vi "AGGIUNGI CARATTERISTICHE GRAFICO.vi"() -> ()   [LabVIEW 2019]
uses:
  TypeDef/Definizione_Grafico_REPORT_OLD.ctl
  TypeDef/Definizione_Grafico_REPORT.ctl
panel:
  out "output cluster":T1={"ASSE X 1"={"NOME ASSE"="", "AUTO\nSCALA?"=FALSE, "MIN"=0.0, "MAX"=0.0, "Colore asse"=0, "Griglie Maggiori"=0, "Griglie Minori"=0, "Decimali"=1}, "ASSE X 2"={"NOME ASSE"="", "AUTO\nSCALA?"=FALSE, "MIN"=0.0, "MAX"=0.0, "Colore asse"=0, "Griglie Maggiori"=0, "Griglie Minori"=0, "Decimali"=1}, "ASSE Y 1"={"NOME ASSE"="", "AUTO\nSCALA?"=FALSE, "MIN"=0.0, "MAX"=0.0, "Colore asse"=0, "Griglie Maggiori"=0, "Griglie Minori"=0, "Decimali"=1}, "ASSE Y 2"={"NOME ASSE"="", "AUTO\nSCALA?"=FALSE, "MIN"=0.0, "MAX"=0.0, "Colore asse"=0, "Griglie Maggiori"=0, "Griglie Minori"=0, "Decimali"=1}, "ASSE Y 3"={"NOME ASSE"="", "AUTO\nSCALA?"=FALSE, "MIN"=0.0, "MAX"=0.0, "Colore asse"=0, "Griglie Maggiori"=0, "Griglie Minori"=0, "Decimali"=1}, "ASSE Y 4"={"NOME ASSE"="", "AUTO\nSCALA?"=FALSE, "MIN"=0.0, "MAX"=0.0, "Colore asse"=0, "Griglie Maggiori"=0, "Griglie Minori"=0, "Decimali"=1}, "X1"=FALSE, "X2"=FALSE, "Y1"=FALSE, "Y2"=FALSE, "Y3"=FALSE, "Y4"=FALSE, "NOME GRAFICO"="", "PROVE ASSOCIATE"={"A FREDDO"=FALSE, "A VUOTO"=FALSE, "A CARICO"=FALSE, "TERMICA"=FALSE, "C.MECC."=FALSE, "ROT BLOCC"=FALSE, "GENERICA"=FALSE, "TABELLA RESISTOMAT"=FALSE, "SCORTA 2"=FALSE, "SCORTA 3"=FALSE}, "ASSE Y 5"={"NOME ASSE"="", "AUTO\nSCALA?"=FALSE, "MIN"=0.0, "MAX"=0.0, "Colore asse"=0, "Griglie Maggiori"=0, "Griglie Minori"=0, "Decimali"=1}, "Y5"=FALSE, "Colore sfondo grafico"=0} {"ASSE Y 5"."Decimali" min=0; "ASSE Y 4"."Decimali" min=0; "ASSE Y 3"."Decimali" min=0; "ASSE Y 2"."Decimali" min=0; "ASSE Y 1"."Decimali" min=0; "ASSE X 2"."Decimali" min=0; "ASSE X 1"."Decimali" min=0}
  in  "file path (use dialog)":path
  out "GRAFICO":T2={"ASSE X 1"={"NOME ASSE"="Time[s]", "AUTO\nSCALA?"=TRUE, "MIN"=0.0, "MAX"=0.0, "Colore asse"=16448250, "Griglie Maggiori"=0, "Griglie Minori"=0}, "ASSE X 2"={"NOME ASSE"="", "AUTO\nSCALA?"=FALSE, "MIN"=0.0, "MAX"=0.0, "Colore asse"=16448250, "Griglie Maggiori"=0, "Griglie Minori"=0}, "ASSE Y 1"={"NOME ASSE"="Voltage[V]", "AUTO\nSCALA?"=TRUE, "MIN"=0.0, "MAX"=0.0, "Colore asse"=16448250, "Griglie Maggiori"=0, "Griglie Minori"=0}, "ASSE Y 2"={"NOME ASSE"="C[Nm]", "AUTO\nSCALA?"=FALSE, "MIN"=0.0, "MAX"=1.0, "Colore asse"=16448250, "Griglie Maggiori"=0, "Griglie Minori"=0}, "ASSE Y 3"={"NOME ASSE"="Pot[kW]", "AUTO\nSCALA?"=FALSE, "MIN"=0.0, "MAX"=0.0, "Colore asse"=16448250, "Griglie Maggiori"=0, "Griglie Minori"=0}, "ASSE Y 4"={"NOME ASSE"="eff[%]", "AUTO\nSCALA?"=FALSE, "MIN"=0.0, "MAX"=0.0, "Colore asse"=16448250, "Griglie Maggiori"=0, "Griglie Minori"=0}, "X1"=TRUE, "X2"=FALSE, "Y1"=TRUE, "Y2"=TRUE, "Y3"=FALSE, "Y4"=FALSE, "NOME GRAFICO"="Voltage-Time 2", "PROVE ASSOCIATE"={"A FREDDO"=FALSE, "A VUOTO"=TRUE, "A CARICO"=FALSE, "TERMICA"=FALSE, "C.MECC."=FALSE, "ROT BLOCC"=FALSE, "GENERICA"=FALSE, "SCORTA 1"=FALSE, "SCORTA 2"=FALSE, "SCORTA 3"=FALSE}, "ASSE Y 5"={"NOME ASSE"="", "AUTO\nSCALA?"=FALSE, "MIN"=0.0, "MAX"=0.0, "Colore asse"=16448250, "Griglie Maggiori"=0, "Griglie Minori"=0}, "Y5"=FALSE, "Colore sfondo grafico"=0}
  out "Array":T2[](array[typedef])
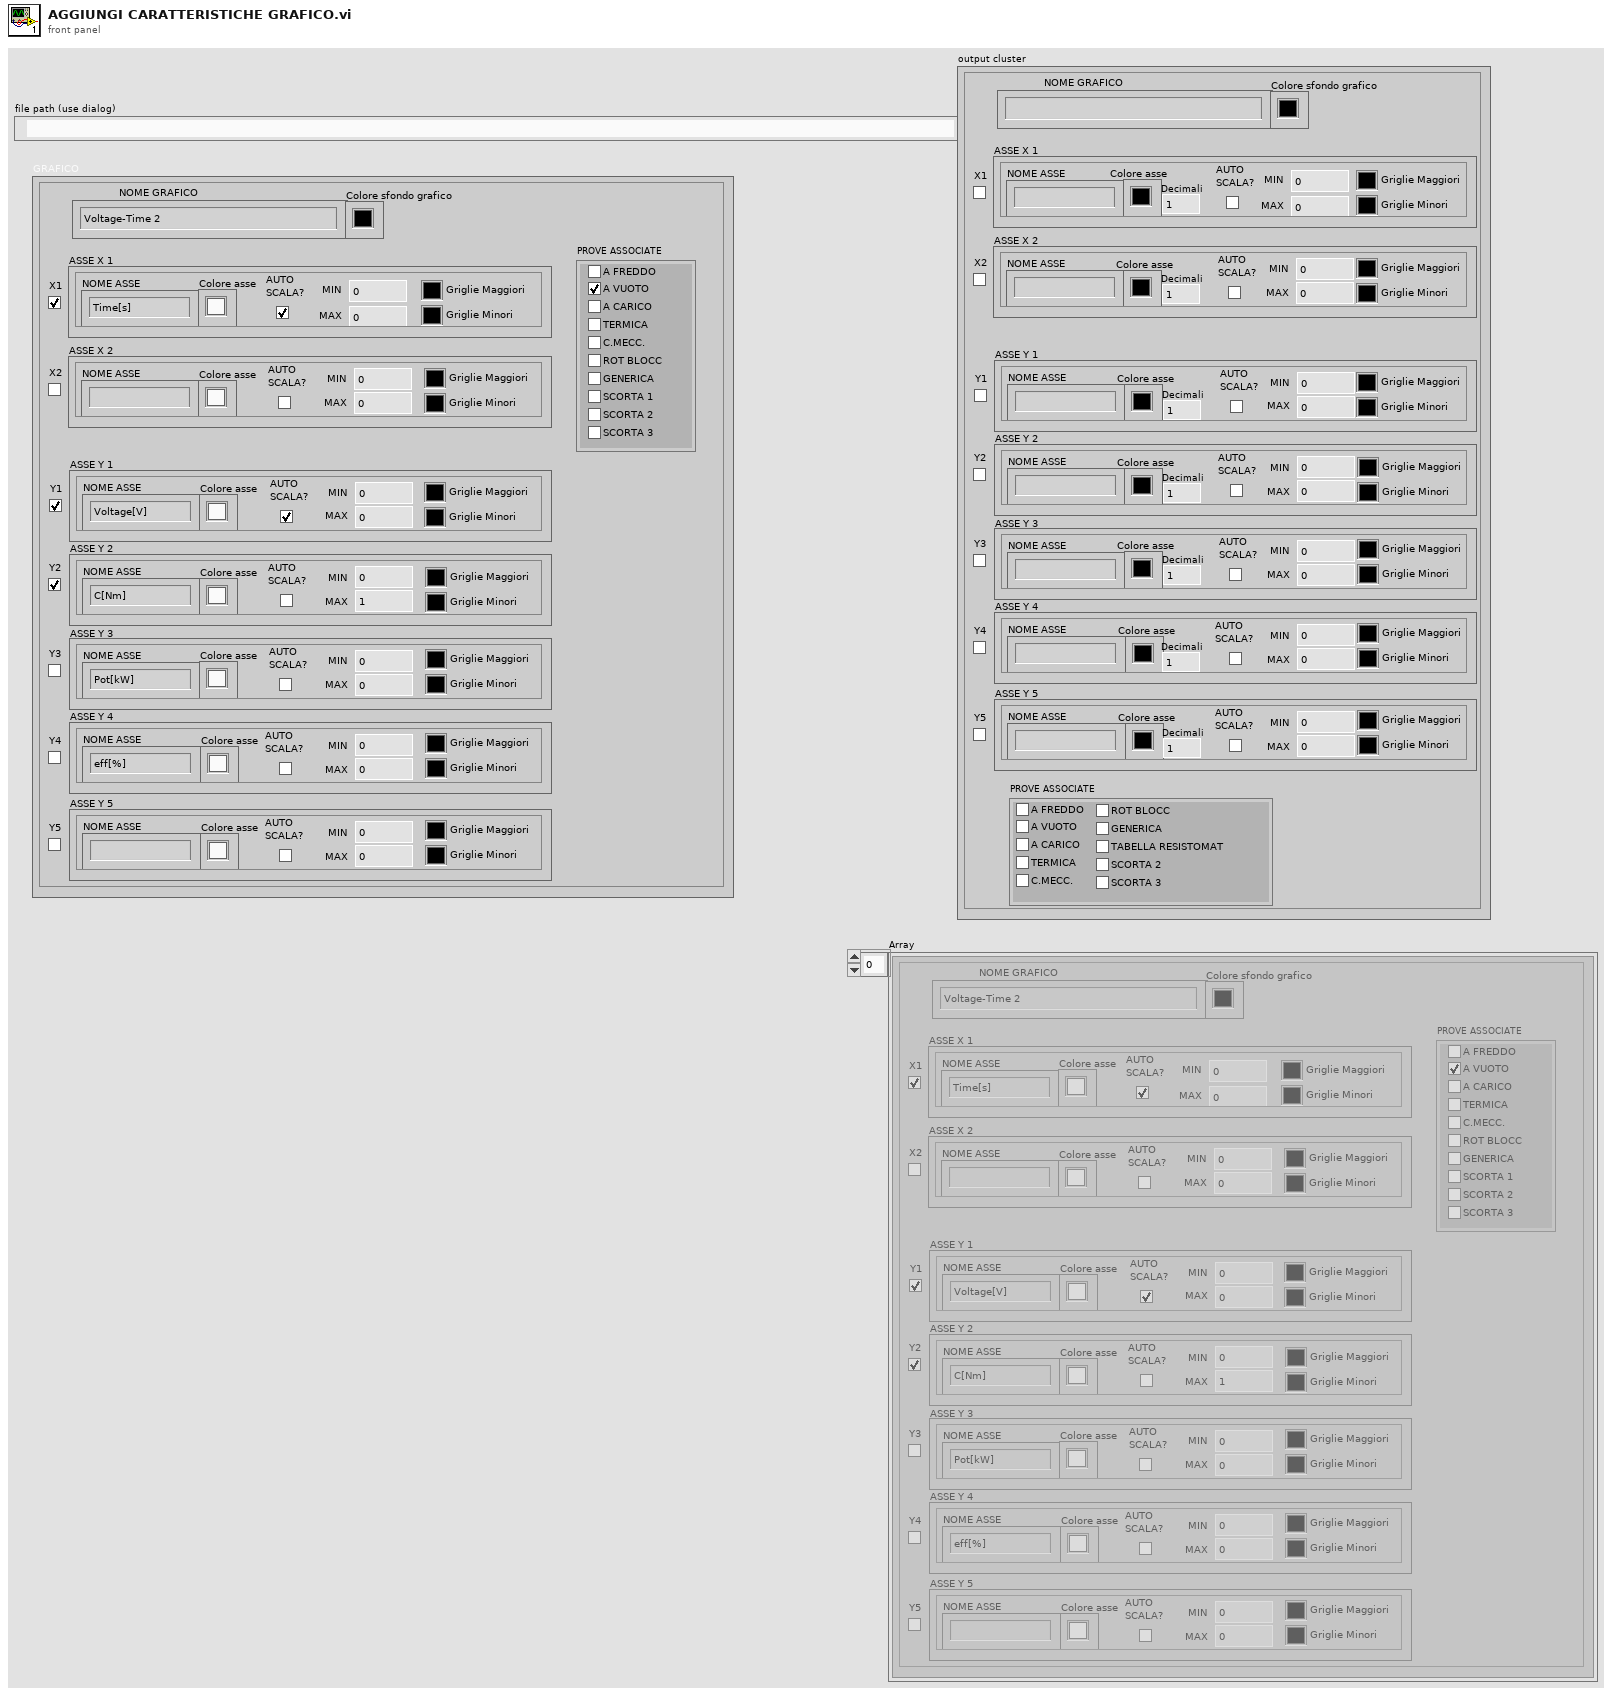
[diagram p1: front panel]
types:
  T1 = typedef "Definizione_Grafico_REPORT.ctl" = cluster{"ASSE X 1":cluster{"NOME ASSE":string, "AUTO\nSCALA?":bool, "MIN":dbl, "MAX":dbl, "Colore asse":u32, "Griglie Maggiori":u32, "Griglie Minori":u32, "Decimali":i8}, "ASSE X 2":cluster{"NOME ASSE":string, "AUTO\nSCALA?":bool, "MIN":dbl, "MAX":dbl, "Colore asse":u32, "Griglie Maggiori":u32, "Griglie Minori":u32, "Decimali":i8}, "ASSE Y 1":cluster{"NOME ASSE":string, "AUTO\nSCALA?":bool, "MIN":dbl, "MAX":dbl, "Colore asse":u32, "Griglie Maggiori":u32, "Griglie Minori":u32, "Decimali":i8}, "ASSE Y 2":cluster{"NOME ASSE":string, "AUTO\nSCALA?":bool, "MIN":dbl, "MAX":dbl, "Colore asse":u32, "Griglie Maggiori":u32, "Griglie Minori":u32, "Decimali":i8}, "ASSE Y 3":cluster{"NOME ASSE":string, "AUTO\nSCALA?":bool, "MIN":dbl, "MAX":dbl, "Colore asse":u32, "Griglie Maggiori":u32, "Griglie Minori":u32, "Decimali":i8}, "ASSE Y 4":cluster{"NOME ASSE":string, "AUTO\nSCALA?":bool, "MIN":dbl, "MAX":dbl, "Colore asse":u32, "Griglie Maggiori":u32, "Griglie Minori":u32, "Decimali":i8}, "X1":bool, "X2":bool, "Y1":bool, "Y2":bool, "Y3":bool, "Y4":bool, "NOME GRAFICO":string, "PROVE ASSOCIATE":cluster{"A FREDDO":bool, "A VUOTO":bool, "A CARICO":bool, "TERMICA":bool, "C.MECC.":bool, "ROT BLOCC":bool, "GENERICA":bool, "TABELLA RESISTOMAT":bool, "SCORTA 2":bool, "SCORTA 3":bool}, "ASSE Y 5":cluster{"NOME ASSE":string, "AUTO\nSCALA?":bool, "MIN":dbl, "MAX":dbl, "Colore asse":u32, "Griglie Maggiori":u32, "Griglie Minori":u32, "Decimali":i8}, "Y5":bool, "Colore sfondo grafico":u32}
  T2 = typedef "Definizione_Grafico_REPORT_OLD.ctl" = cluster{"ASSE X 1":cluster{"NOME ASSE":string, "AUTO\nSCALA?":bool, "MIN":dbl, "MAX":dbl, "Colore asse":u32, "Griglie Maggiori":u32, "Griglie Minori":u32}, "ASSE X 2":cluster{"NOME ASSE":string, "AUTO\nSCALA?":bool, "MIN":dbl, "MAX":dbl, "Colore asse":u32, "Griglie Maggiori":u32, "Griglie Minori":u32}, "ASSE Y 1":cluster{"NOME ASSE":string, "AUTO\nSCALA?":bool, "MIN":dbl, "MAX":dbl, "Colore asse":u32, "Griglie Maggiori":u32, "Griglie Minori":u32}, "ASSE Y 2":cluster{"NOME ASSE":string, "AUTO\nSCALA?":bool, "MIN":dbl, "MAX":dbl, "Colore asse":u32, "Griglie Maggiori":u32, "Griglie Minori":u32}, "ASSE Y 3":cluster{"NOME ASSE":string, "AUTO\nSCALA?":bool, "MIN":dbl, "MAX":dbl, "Colore asse":u32, "Griglie Maggiori":u32, "Griglie Minori":u32}, "ASSE Y 4":cluster{"NOME ASSE":string, "AUTO\nSCALA?":bool, "MIN":dbl, "MAX":dbl, "Colore asse":u32, "Griglie Maggiori":u32, "Griglie Minori":u32}, "X1":bool, "X2":bool, "Y1":bool, "Y2":bool, "Y3":bool, "Y4":bool, "NOME GRAFICO":string, "PROVE ASSOCIATE":cluster{"A FREDDO":bool, "A VUOTO":bool, "A CARICO":bool, "TERMICA":bool, "C.MECC.":bool, "ROT BLOCC":bool, "GENERICA":bool, "SCORTA 1":bool, "SCORTA 2":bool, "SCORTA 3":bool}, "ASSE Y 5":cluster{"NOME ASSE":string, "AUTO\nSCALA?":bool, "MIN":dbl, "MAX":dbl, "Colore asse":u32, "Griglie Maggiori":u32, "Griglie Minori":u32}, "Y5":bool, "Colore sfondo grafico":u32}
  T3 = enum16{"open", "replace", "create", "open or create", "replace or create", "replace or create with confirmation"}
  T4 = cluster{"A FREDDO":bool, "A VUOTO":bool, "A CARICO":bool, "TERMICA":bool, "C.MECC.":bool, "ROT BLOCC":bool, "GENERICA":bool, "SCORTA 1":bool, "SCORTA 2":bool, "SCORTA 3":bool}
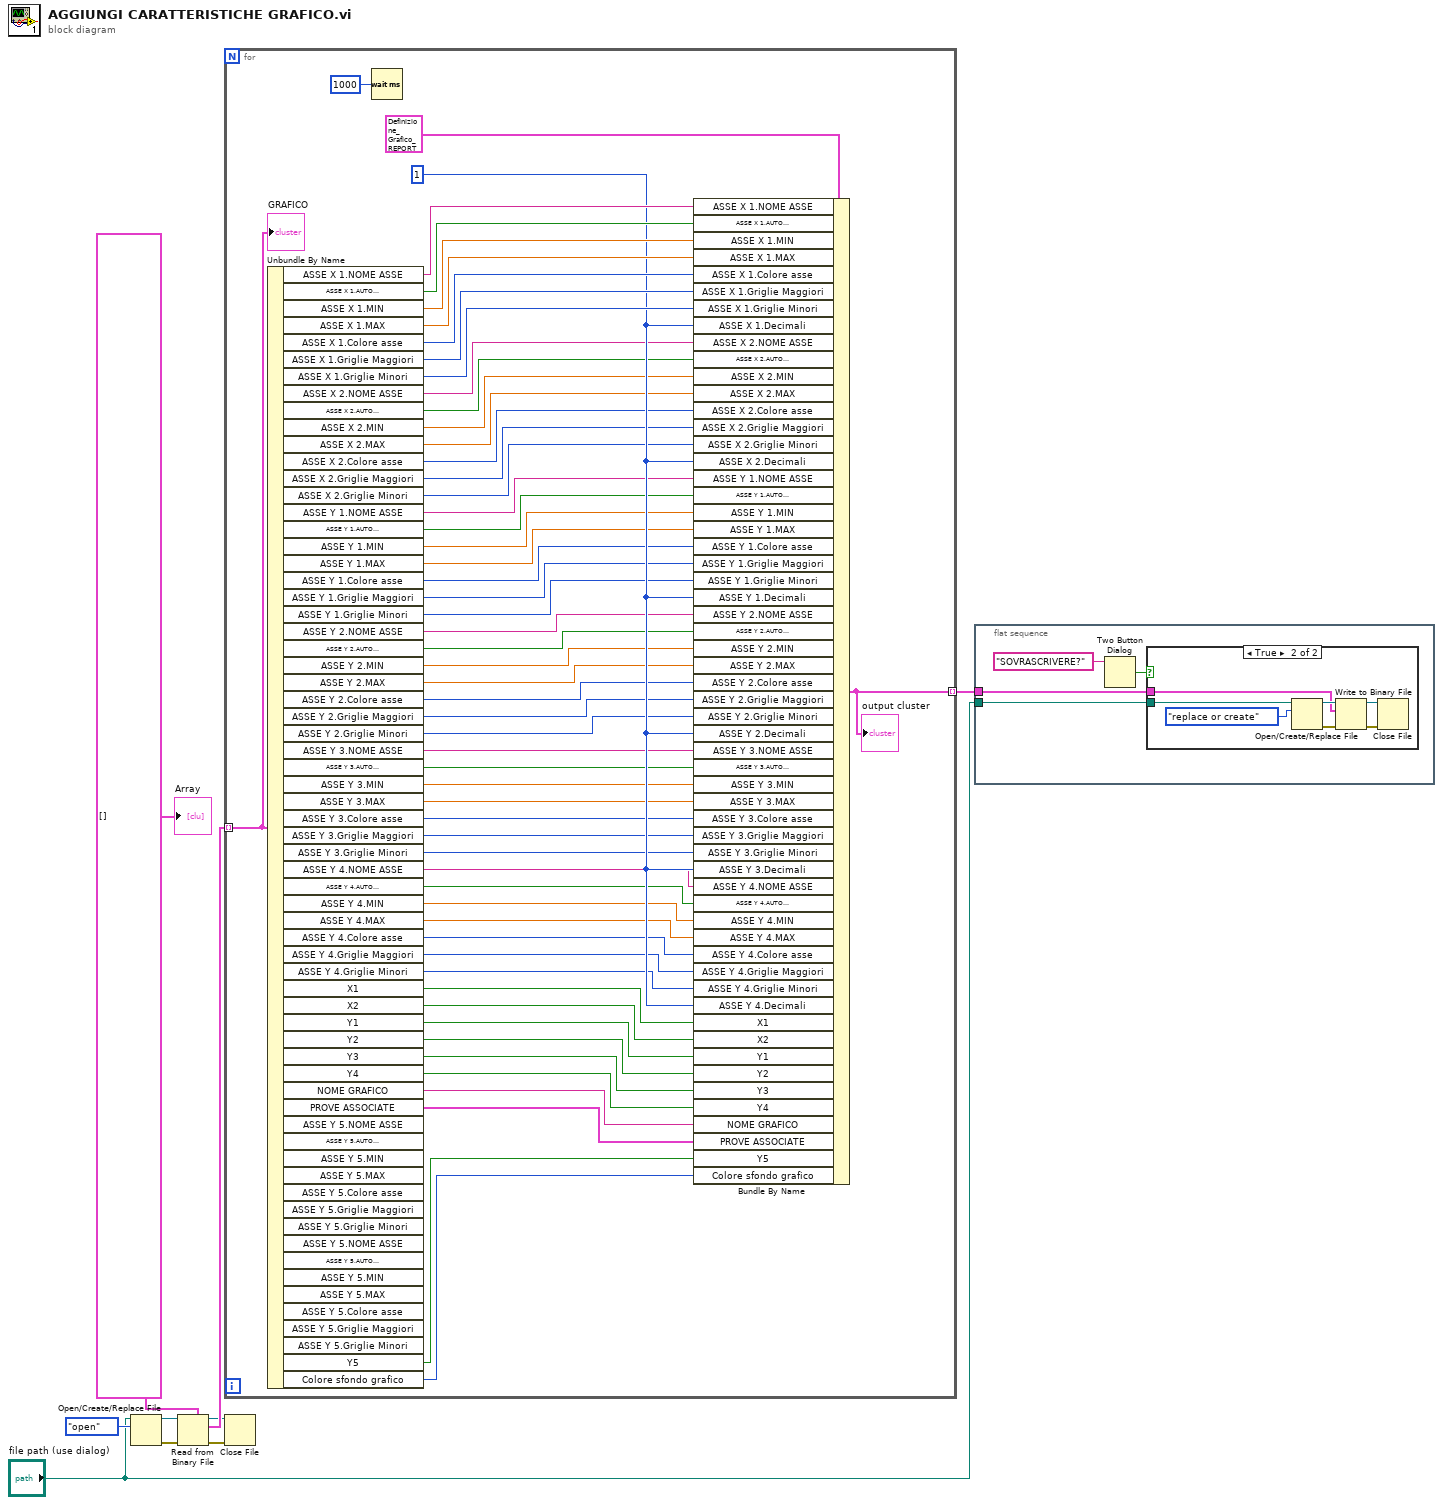
[diagram p0: block diagram]
diagram:
  w5 = T2[] []
  n1 = Open/Create/Replace File(file path (use dialog)="file path (use dialog)", operation (0:open)=T3."open") -> (refnum out=w8:refnum<file>, error out=w9:errorcluster)  [unwired: 4 in, 1 out]
  n2 = Read from Binary File(5:w5, 8:w9, 11:w8) -> (0:w3:errorcluster, 2:w6:T2[], 3:w4:refnum<file>)  [unwired: 3 in, 1 out]
  n3 = for {
    tunnel: w6 -> [w11] mode=indexing
    tunnel: [w12] -> w1 mode=indexing
    w58 = 1
    n4 = Unbundle By Name(w11) -> ("ASSE X 1.NOME ASSE"=w65:string, "ASSE X 1.AUTO\nSCALA?"=w64:bool, "ASSE X 1.MIN"=w63:dbl, "ASSE X 1.MAX"=w62:dbl, "ASSE X 1.Colore asse"=w61:u32, "ASSE X 1.Griglie Maggiori"=w60:u32, "ASSE X 1.Griglie Minori"=w59:u32, "ASSE X 2.NOME ASSE"=w57:string, "ASSE X 2.AUTO\nSCALA?"=w56:bool, "ASSE X 2.MIN"=w55:dbl, "ASSE X 2.MAX"=w54:dbl, "ASSE X 2.Colore asse"=w53:u32, "ASSE X 2.Griglie Maggiori"=w52:u32, "ASSE X 2.Griglie Minori"=w51:u32, "ASSE Y 1.NOME ASSE"=w50:string, "ASSE Y 1.AUTO\nSCALA?"=w49:bool, "ASSE Y 1.MIN"=w48:dbl, "ASSE Y 1.MAX"=w47:dbl, "ASSE Y 1.Colore asse"=w46:u32, "ASSE Y 1.Griglie Maggiori"=w45:u32, "ASSE Y 1.Griglie Minori"=w44:u32, "ASSE Y 2.NOME ASSE"=w43:string, "ASSE Y 2.AUTO\nSCALA?"=w42:bool, "ASSE Y 2.MIN"=w41:dbl, "ASSE Y 2.MAX"=w40:dbl, "ASSE Y 2.Colore asse"=w39:u32, "ASSE Y 2.Griglie Maggiori"=w38:u32, "ASSE Y 2.Griglie Minori"=w37:u32, "ASSE Y 3.NOME ASSE"=w36:string, "ASSE Y 3.AUTO\nSCALA?"=w35:bool, "ASSE Y 3.MIN"=w34:dbl, "ASSE Y 3.MAX"=w33:dbl, "ASSE Y 3.Colore asse"=w32:u32, "ASSE Y 3.Griglie Maggiori"=w31:u32, "ASSE Y 3.Griglie Minori"=w30:u32, "ASSE Y 4.NOME ASSE"=w29:string, "ASSE Y 4.AUTO\nSCALA?"=w28:bool, "ASSE Y 4.MIN"=w27:dbl, "ASSE Y 4.MAX"=w26:dbl, "ASSE Y 4.Colore asse"=w25:u32, "ASSE Y 4.Griglie Maggiori"=w24:u32, "ASSE Y 4.Griglie Minori"=w23:u32, "X1"=w22:bool, "X2"=w21:bool, "Y1"=w20:bool, "Y2"=w19:bool, "Y3"=w18:bool, "Y4"=w17:bool, "NOME GRAFICO"=w16:string, "PROVE ASSOCIATE"=w15:T4, "Y5"=w14:bool, "Colore sfondo grafico"=w13:u32)  [unwired: 14 out]
    n5 = Wait (ms)(milliseconds to wait=u32 1000) -> ()  [unwired: 1 out]
    n6 = Bundle By Name(cluster=T1 {"ASSE X 1"={"NOME ASSE"="", "AUTO\nSCALA?"=FALSE, "MIN"=0.0, "MAX"=0.0, "Colore asse"=0, "Griglie Maggiori"=0, "Griglie Minori"=0, "Decimali"=1}, "ASSE X 2"={"NOME ASSE"="", "AUTO\nSCALA?"=FALSE, "MIN"=0.0, "MAX"=0.0, "Colore asse"=0, "Griglie Maggiori"=0, "Griglie Minori"=0, "Decimali"=1}, "ASSE Y 1"={"NOME ASSE"="", "AUTO\nSCALA?"=FALSE, "MIN"=0.0, "MAX"=0.0, "Colore asse"=0, "Griglie Maggiori"=0, "Griglie Minori"=0, "Decimali"=1}, "ASSE Y 2"={"NOME ASSE"="", "AUTO\nSCALA?"=FALSE, "MIN"=0.0, "MAX"=0.0, "Colore asse"=0, "Griglie Maggiori"=0, "Griglie Minori"=0, "Decimali"=1}, "ASSE Y 3"={"NOME ASSE"="", "AUTO\nSCALA?"=FALSE, "MIN"=0.0, "MAX"=0.0, "Colore asse"=0, "Griglie Maggiori"=0, "Griglie Minori"=0, "Decimali"=1}, "ASSE Y 4"={"NOME ASSE"="", "AUTO\nSCALA?"=FALSE, "MIN"=0.0, "MAX"=0.0, "Colore asse"=0, "Griglie Maggiori"=0, "Griglie Minori"=0, "Decimali"=1}, "X1"=TRUE, "X2"=TRUE, "Y1"=TRUE, "Y2"=TRUE, "Y3"=TRUE, "Y4"=TRUE, "NOME GRAFICO"="", "PROVE ASSOCIATE"={"A FREDDO"=FALSE, "A VUOTO"=FALSE, "A CARICO"=FALSE, "TERMICA"=FALSE, "C.MECC."=FALSE, "ROT BLOCC"=FALSE, "GENERICA"=FALSE, "TABELLA RESISTOMAT"=FALSE, "SCORTA 2"=FALSE, "SCORTA 3"=FALSE}, "ASSE Y 5"={"NOME ASSE"="", "AUTO\nSCALA?"=FALSE, "MIN"=0.0, "MAX"=0.0, "Colore asse"=0, "Griglie Maggiori"=0, "Griglie Minori"=0, "Decimali"=1}, "Y5"=FALSE, "Colore sfondo grafico"=0} ("GRAFICO 2"), "ASSE X 1.NOME ASSE"=w65, "ASSE X 1.AUTO\nSCALA?"=w64, "ASSE X 1.MIN"=w63, "ASSE X 1.MAX"=w62, "ASSE X 1.Colore asse"=w61, "ASSE X 1.Griglie Maggiori"=w60, "ASSE X 1.Griglie Minori"=w59, "ASSE X 1.Decimali"=w58, "ASSE X 2.NOME ASSE"=w57, "ASSE X 2.AUTO\nSCALA?"=w56, "ASSE X 2.MIN"=w55, "ASSE X 2.MAX"=w54, "ASSE X 2.Colore asse"=w53, "ASSE X 2.Griglie Maggiori"=w52, "ASSE X 2.Griglie Minori"=w51, "ASSE X 2.Decimali"=w58, "ASSE Y 1.NOME ASSE"=w50, "ASSE Y 1.AUTO\nSCALA?"=w49, "ASSE Y 1.MIN"=w48, "ASSE Y 1.MAX"=w47, "ASSE Y 1.Colore asse"=w46, "ASSE Y 1.Griglie Maggiori"=w45, "ASSE Y 1.Griglie Minori"=w44, "ASSE Y 1.Decimali"=w58, "ASSE Y 2.NOME ASSE"=w43, "ASSE Y 2.AUTO\nSCALA?"=w42, "ASSE Y 2.MIN"=w41, "ASSE Y 2.MAX"=w40, "ASSE Y 2.Colore asse"=w39, "ASSE Y 2.Griglie Maggiori"=w38, "ASSE Y 2.Griglie Minori"=w37, "ASSE Y 2.Decimali"=w58, "ASSE Y 3.NOME ASSE"=w36, "ASSE Y 3.AUTO\nSCALA?"=w35, "ASSE Y 3.MIN"=w34, "ASSE Y 3.MAX"=w33, "ASSE Y 3.Colore asse"=w32, "ASSE Y 3.Griglie Maggiori"=w31, "ASSE Y 3.Griglie Minori"=w30, "ASSE Y 3.Decimali"=w58, "ASSE Y 4.NOME ASSE"=w29, "ASSE Y 4.AUTO\nSCALA?"=w28, "ASSE Y 4.MIN"=w27, "ASSE Y 4.MAX"=w26, "ASSE Y 4.Colore asse"=w25, "ASSE Y 4.Griglie Maggiori"=w24, "ASSE Y 4.Griglie Minori"=w23, "ASSE Y 4.Decimali"=w58, "X1"=w22, "X2"=w21, "Y1"=w20, "Y2"=w19, "Y3"=w18, "Y4"=w17, "NOME GRAFICO"=w16, "PROVE ASSOCIATE"=w15, "Y5"=w14, "Colore sfondo grafico"=w13) -> (w12:T1)
    "output cluster" <- w12
    "GRAFICO" <- w11
  }
  n7 = Close File(refnum=w4, error in=w3) -> ()  [unwired: 2 out]
  n8 = flat-sequence {
    tunnel: "file path (use dialog)" -> [w70]
    tunnel: w1 -> [w67]
    frame #0 {
      n9 = Two Button Dialog(message="SOVRASCRIVERE?") -> (T button?=w69:bool)  [unwired: 2 in]
      n10 = case shown="True" w69 {
        tunnel: w70 -> [_ w72]
        tunnel: w67 -> [_ w71]
        frame False {
        }
        frame True {
          n11 = Open/Create/Replace File(file path (use dialog)=w72, operation (0:open)=T3."replace or create") -> (refnum out=w76:refnum<file>, error out=w77:errorcluster)  [unwired: 4 in, 1 out]
          n12 = Write to Binary File(file (use dialog)=w76, data=w71, error in=w77) -> (refnum out=w73:refnum<file>, error out=w74:errorcluster)  [unwired: 3 in, 1 out]
          n13 = Close File(refnum=w73, error in=w74) -> ()  [unwired: 2 out]
        }
      }
    }
  }
  "Array" <- w5
